vi "freqgammabox.vi"(5 "aggregator action":T1, 7 "buffer size":i32=100, 9 "Gamma (Hz)":dbl=0.1 format="%#_10f", 10 "freq (Hz)":dbl=0.1 format="%#_10f") -> (1 "gamma OUT (Hz)":dbl=0.1 format="%#_10f", 2 "freq OUT (Hz)":dbl=0.1 format="%#_10f")   [LabVIEW 2020]
uses:
  agregator -- action.ctl
  interpolation state - real.ctl
  linear interpolation - real.vi
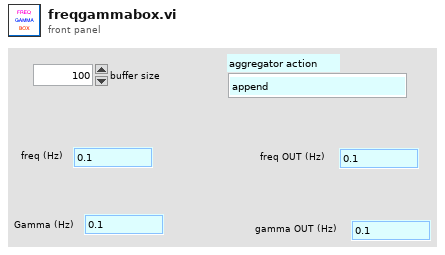
[diagram p1: front panel]
types:
  T1 = typedef "agregator -- action.ctl" = enum16{"append", "interpolate", "empty!", "force", "init", "scale", "read last"}
  T2 = typedef "interpolation state - real.ctl" = cluster{"requested size":i32, "Array":dbl[], "actual number of elements":i32}
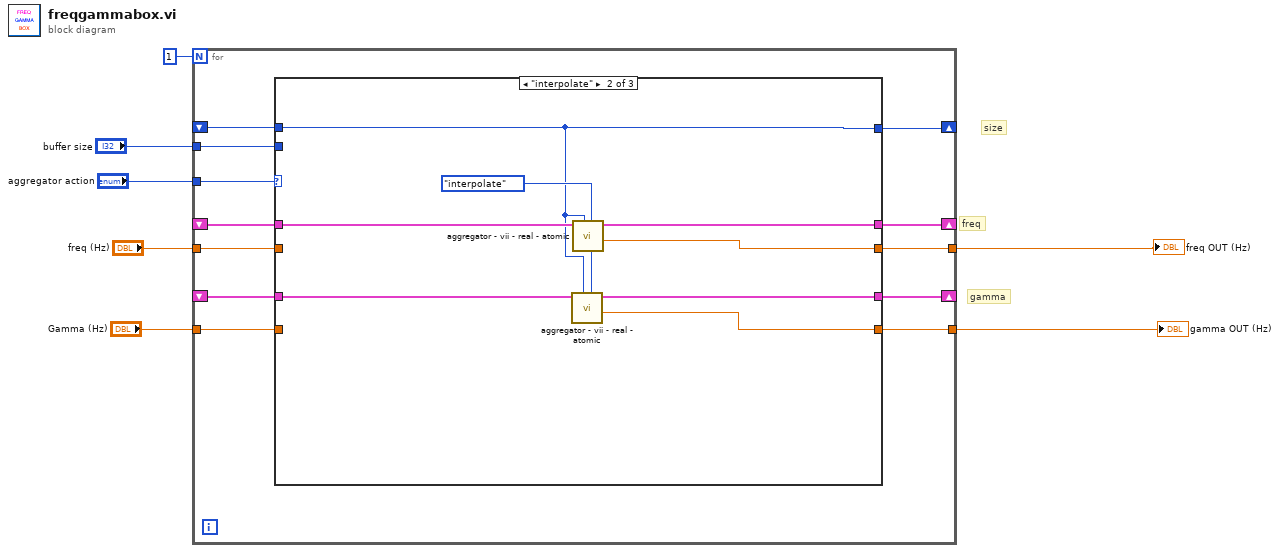
[diagram p0: block diagram]
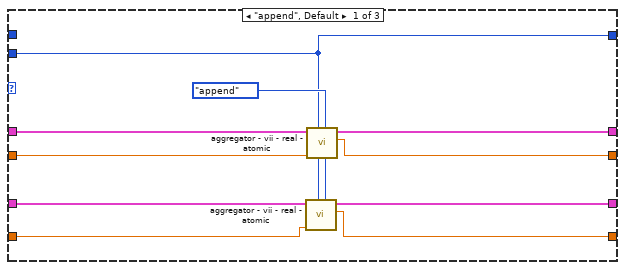
[diagram p2: hidden frame]
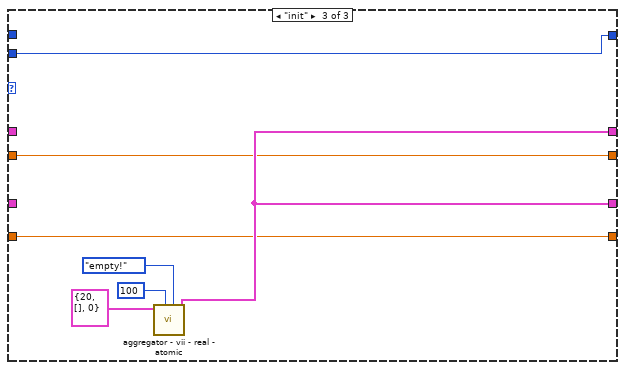
[diagram p3: hidden frame]
diagram:
  # "size"
  # "gamma"
  # "freq"
  n1 = for {
    N: 1 -> [_]
    tunnel: "aggregator action" -> [w19]
    shift-right: [w18] -> _
    shift-left: _ -> [w15]
    shift-right: [w17] -> _
    shift-left: _ -> [w14]
    tunnel: "buffer size" -> [w16]
    tunnel: "freq (Hz)" -> [w13]
    tunnel: "Gamma (Hz)" -> [w12]
    shift-right: [w11] -> _
    shift-left: _ -> [w10]
    tunnel: [w9] -> w1
    tunnel: [w8] -> w2
    n2 = case shown="\"interpolate\"" w19 {
      tunnel: [w27 w35 w41] -> w18
      tunnel: [w25 w33 w41] -> w17
      tunnel: w16 -> [w22 _ w40]
      tunnel: w15 -> [w28 w36 _]
      tunnel: w14 -> [w26 w34 _]
      tunnel: w13 -> [w24 _ w39]
      tunnel: w12 -> [w23 _ w38]
      tunnel: [w22 w32 w40] -> w11
      tunnel: w10 -> [_ w32 _]
      tunnel: [w21 w31 w39] -> w9
      tunnel: [w20 w30 w38] -> w8
      frame "append", Default {
        w29 = agregator_--_action."append" ("aggregator action")
        n3 = call "aggregator - vii - real - atomic.vi"("aggregator action"=w29, "requested size"=w22, "number"=w23, "state IN"=w26) -> ("mean"=w20:dbl, "state OUT"=w25:T2)  [unwired: 4 in, 2 out]
        n4 = call "aggregator - vii - real - atomic.vi"("aggregator action"=w29, "requested size"=w22, "number"=w24, "state IN"=w28) -> ("mean"=w21:dbl, "state OUT"=w27:T2)  [unwired: 4 in, 2 out]
      }
      frame "interpolate" {
        w37 = agregator_--_action."interpolate" ("aggregator action")
        n5 = call "aggregator - vii - real - atomic.vi"("aggregator action"=w37, "requested size"=w32, "state IN"=w34) -> ("interp average"=w30:dbl, "state OUT"=w33:T2)  [unwired: 5 in, 2 out]
        n6 = call "aggregator - vii - real - atomic.vi"("aggregator action"=w37, "requested size"=w32, "state IN"=w36) -> ("interp average"=w31:dbl, "state OUT"=w35:T2)  [unwired: 5 in, 2 out]
      }
      frame "init" {
        n7 = call "aggregator - vii - real - atomic.vi"("aggregator action"=agregator_--_action."empty!", "requested size"=100, "state IN"=T2 {"requested size"=20, "Array"=[], "actual number of elements"=0}) -> ("state OUT"=w41:T2)  [unwired: 5 in, 3 out]
      }
    }
  }
  "freq OUT (Hz)" <- w1
  "gamma OUT (Hz)" <- w2
